vi "Report_Type.vi"(8 "error in (no error)":errorcluster, 11 "IB_SDIST in":refnum<class "IB_SDIST.lvclass">) -> (0 "error out":errorcluster, 2 "type":string, 3 "IB_SDIST out":refnum<class "IB_SDIST.lvclass">)   [LabVIEW 2020, in "IB_SDIST.lvclass"]
uses:
  <vilib>/AppBuilder/IB_Classes/Source/Container/Build/SDIST/IB_SDIST.lvclass
  <vilib>/AppBuilder/IB_Classes/Source/Container/Build/SDIST/IB_SDIST.lvclass/IB_SDIST.ctl
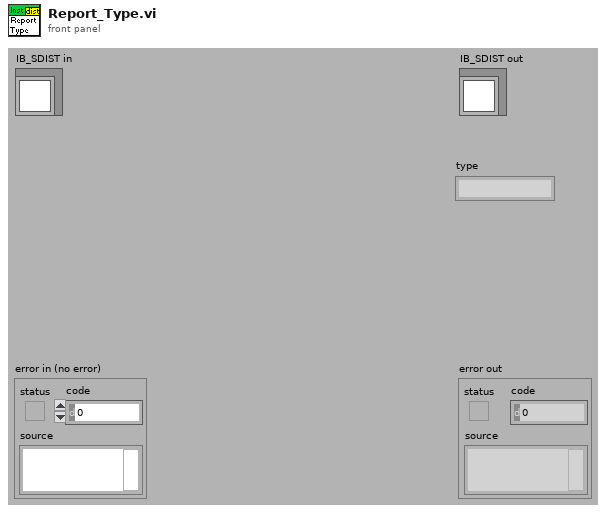
[diagram p1: front panel]
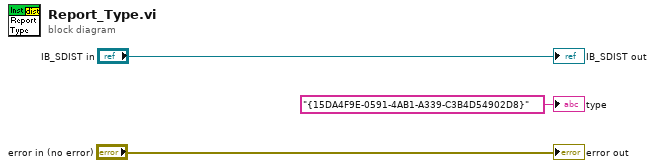
[diagram p0: block diagram]
diagram:
  "error out" <- "error in (no error)"
  "IB_SDIST out" <- "IB_SDIST in"
  "type" <- "{15DA4F9E-0591-4AB1-A339-C3B4D54902D8}" ("type")
